vi "Flatten repeated.vi"(7 "Field Number":i32, 10 "Data":T1[](array[typedef]), 11 "Buffer in":u8[](array[numeric]) format="%.0x") -> (3 "Buffer":u8[](array[numeric]) format="%.0x")   [LabVIEW 2020, in "Service.lvlib"]
uses:
  Service.lvlib
  Data.ctl
  lv-protoc/LV-Proto/Wire Encode Tag.vi
  lv-protoc/LV-Proto/Encode LEN.vi
  lv-protoc/LV-Proto/Wire Encode Varint I32.vi
  lv-protoc/LV-Proto/LV-Proto.lvlib
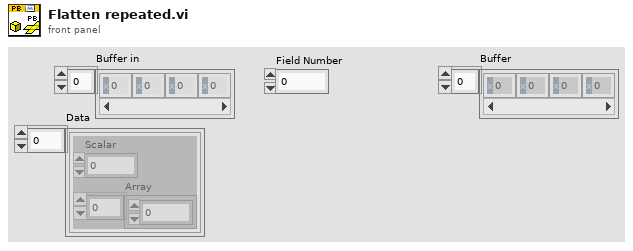
[diagram p1: front panel]
types:
  T1 = typedef "Service.lvlib/Data.ctl" = cluster{"Scalar":dbl, "Array":dbl[]}
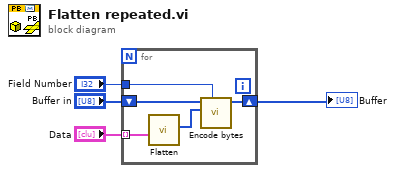
[diagram p0: block diagram]
diagram:
  n1 = for {
    shift-right: [w7] -> w3
    shift-left: "Buffer in" -> [w9]
    tunnel: "Data" -> [w5] mode=indexing
    tunnel: "Field Number" -> [w6]
    n2 = call "Flatten.vi"("Data"=w5) -> ("Buffer"=w8:u8[])  [unwired: 9 in, 1 out]
    n3 = call "Encode bytes.vi"("Field Number"=w6, "bytes"=w8, "Buffer in"=w9) -> ("Buffer"=w7:u8[])  [unwired: 8 in]
  }
  "Buffer" <- w3
